vi "Error 5010 - Empty or Relative Path.vi"() -> (0 "error out":errorcluster)   [LabVIEW 2021]
doc: "Error 5004 - TCP Timeout"
uses:
  <vilib>/Utility/error.llb/Error Cluster From Error Code.vi
  <vilib>/ErrorRing/Error Ring.xnode
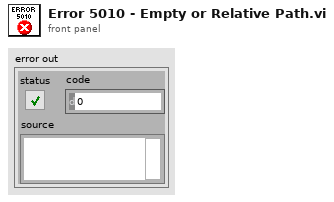
[diagram p1: front panel]
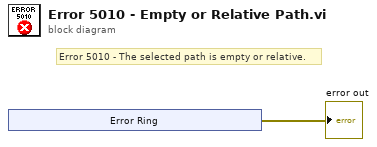
[diagram p0: block diagram]
diagram:
  # "Error 5010 - The selected path is empty or relative."
  n1 = xnode "Error Ring"() -> ("error out"=→"error out":errorcluster)
